vi "LED and dc motor control by the for loop.vi"() -> ()   [LabVIEW 2019]
uses:
  <vilib>/LabVIEW Interface for Arduino/Type Defs/Board Type.ctl
  <vilib>/LabVIEW Interface for Arduino/Type Defs/Connection Type.ctl
  <vilib>/LabVIEW Interface for Arduino/Type Defs/Pin Mode.ctl
  <vilib>/LabVIEW Interface for Arduino/LabVIEW Interface for Arduino.lvlib
panel:
  in  "stop":bool
  in  "VISA resource":refnum<visa-resource-name>
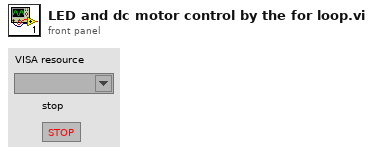
[diagram p1: front panel]
types:
  T1 = typedef "LabVIEW Interface for Arduino.lvlib/Pin Mode.ctl" = enum8{"Input", "Output"}
  T2 = typedef "LabVIEW Interface for Arduino.lvlib/Connection Type.ctl" = enum8{"USB / Serial", "XBEE", "BlueSmirf (Bluetooth)"}
  T3 = typedef "LabVIEW Interface for Arduino.lvlib/Board Type.ctl" = enum16{"Uno", "Dimuelanove w/Atmega 328", "Mega 2560"}
  T4 = typedef "LabVIEW Interface for Arduino.lvlib/Arduino Resource.ctl" = cluster{"VISA resource":refnum<visa-resource-name>, "Board Type":T3, "Connection Type":enum8{"USB / Serial"}, "Bytes Per Packet (15)":u8}
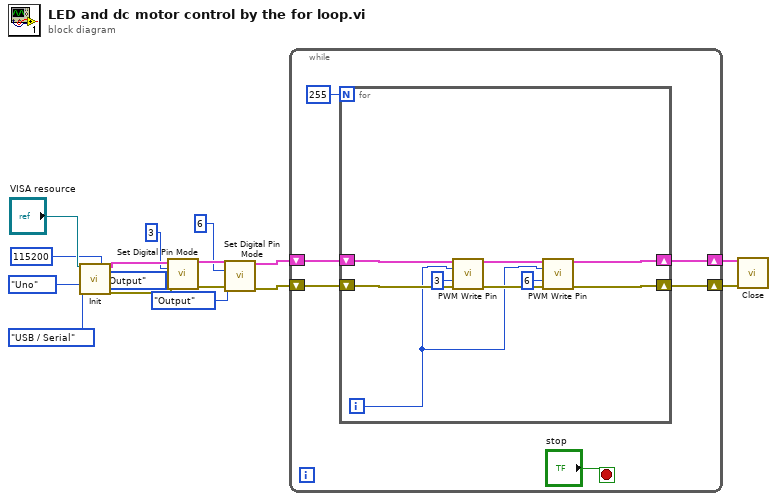
[diagram p0: block diagram]
diagram:
  n1 = call <vilib>:"Init.vi"("VISA resource"="VISA resource", "Baud Rate (115200)"=u32 115200, "Board Type (Uno)"=Board_Type."Uno", "Connection Type (USB/Serial)"=Connection_Type."USB / Serial") -> ("Arduino Resource"=w12:T4, "error out"=w10:errorcluster)  [unwired: 14 in]
  n2 = call <vilib>:"Set Digital Pin Mode.vi"("Arduino Resource"=w12, "Digital I/O Pin"=u8 3, "Pin Mode (Input)"=Pin_Mode."Output", "error in"=w10) -> ("Arduino Resource"=w11:T4, "error out"=w9:errorcluster)  [unwired: 10 in]
  n3 = call <vilib>:"Set Digital Pin Mode.vi"("Arduino Resource"=w11, "Digital I/O Pin"=u8 6, "Pin Mode (Input)"=Pin_Mode."Output", "error in"=w9) -> ("Arduino Resource"=w4:T4, "error out"=w3:errorcluster)  [unwired: 10 in]
  n4 = while {
    shift-right: [w20] -> w2
    shift-left: w4 -> [w22]
    shift-right: [w19] -> w1
    shift-left: w3 -> [w21]
    stop <- "stop" stop-if-true
    n5 = for {
      N: 255 -> [_]
      shift-right: [w27] -> w20
      shift-left: w22 -> [w29]
      shift-right: [w26] -> w19
      shift-left: w21 -> [w28]
      i -> [w23]
      n6 = call <vilib>:"PWM Write Pin.vi"("Arduino Resource"=w29, "Duty Cycle (0 - 255)"=w23, "PWM Pin (3)"=u8 3, "error in"=w28) -> ("Arduino Resource"=w31:T4, "error out"=w30:errorcluster)  [unwired: 10 in]
      n7 = call <vilib>:"PWM Write Pin.vi"("Arduino Resource"=w31, "Duty Cycle (0 - 255)"=w23, "PWM Pin (3)"=u8 6, "error in"=w30) -> ("Arduino Resource"=w27:T4, "error out"=w26:errorcluster)  [unwired: 10 in]
    }
  }
  n8 = call <vilib>:"Close.vi"("Arduino Resource"=w2, "error in"=w1) -> ()  [unwired: 13 in, 1 out]
